vi "Check Solution.vi"() -> ()   [LabVIEW 2013]
panel:
  in  "Schedule 1":i32[](array[numeric])
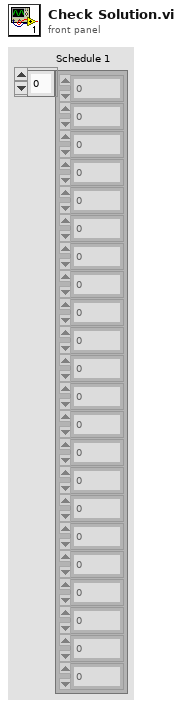
[diagram p1: front panel]
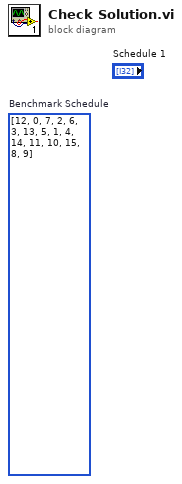
[diagram p0: block diagram]
diagram:
  (unwired) i32[] [12, 0, 7, 2, 6, 3, 13, 5, 1, 4, 14, 11, 10, 15, 8, 9]  # Benchmark Schedule
